vi "Breakfast Menu W3.vi"() -> ()   [LabVIEW 2019, in "Tree Map.lvlib"]
doc: "<b>Author:</b> Piotr Kruczkowski <PrimaryKey>\n<b>License:</b> NewBSD\n\nCopyright (c) 2019, National Instruments\nAll rights reserved.\n\nRedistribution and use in source and binary forms, with or without\nmodification, are permitted provided that the following conditions are met:\n1. Redistributions of source code must retain the above copyright\n notice, this list of conditions and the following disclaimer.\n2. Redistributions in binary form must reproduce the above copyright\n notice, this list of conditions and the following disclaimer in the\n documentation and/or other materials provided with the distribution.\n3. Neither the name of National Instruments nor the\n names of its contributors may be used to endorse or promote products\n derived from this software without specific prior written permission.\n\nTHIS SOFTWARE IS PROVIDED BY National Instruments ''AS IS'' AND ANY\nEXPRESS OR IMPLIED WARRANTIES, INCLUDING, BUT NOT LIMITED TO, THE IMPLIED\nWARRANTIES OF MERCHANTABILITY AND FITNESS FOR A PARTICULAR PURPOSE ARE\nDISCLAIMED. IN NO EVENT SHALL National Instruments BE LIABLE FOR ANY\nDIRECT, INDIRECT, INCIDENTAL, SPECIAL, EXEMPLARY, OR CONSEQUENTIAL DAMAGES\n(INCLUDING, BUT NOT LIMITED TO, PROCUREMENT OF SUBSTITUTE GOODS OR SERVICES;\nLOSS OF USE, DATA, OR PROFITS; OR BUSINESS INTERRUPTION) HOWEVER CAUSED AND\nON ANY THEORY OF LIABILITY, WHETHER IN CONTRACT, STRICT LIABILITY, OR TORT\n(INCLUDING NEGLIGENCE OR OTHERWISE) ARISING IN ANY WAY OUT OF THE USE OF THIS\nSOFTWARE, EVEN IF ADVISED OF THE POSSIBILITY OF SUCH DAMAGE."
uses:
  Tree Map.lvlib
  Tree Map Data.ctl
  API/List Roots.vi
  Utility/Into Tree Control Items.vi
panel:
  out "Tree Map":T1={"\\breakfast_menu"={"Child Paths Set"={"\\breakfast_menu\\food", "\\breakfast_menu\\food_000000", "\\breakfast_menu\\food_000001", "\\breakfast_menu\\food_000002", "\\breakfast_menu\\food_000003"}, "Name"="breakfast_menu", "Data"="", "Attributes"={}}, "\\breakfast_menu\\food"={"Child Paths Set"={"\\breakfast_menu\\food\\calories", "\\breakfast_menu\\food\\description", "\\breakfast_menu\\food\\name", "\\breakfast_menu\\food\\price"}, "Name"="food", "Data"="", "Attributes"={}}, "\\breakfast_menu\\food\\calories"={"Child Paths Set"={}, "Name"="calories", "Data"="650", "Attributes"={}}, "\\breakfast_menu\\food\\description"={"Child Paths Set"={}, "Name"="description", "Data"="Two of our famous Belgian Waffles with plenty of real maple syrup", "Attributes"={}}, "\\breakfast_menu\\food\\name"={"Child Paths Set"={}, "Name"="name", "Data"="Belgian Waffles", "Attributes"={}}, "\\breakfast_menu\\food\\price"={"Child Paths Set"={}, "Name"="price", "Data"="$5.95", "Attributes"={}}, "\\breakfast_menu\\food_000000"={"Child Paths Set"={"\\breakfast_menu\\food_000000\\calories", "\\breakfast_menu\\food_000000\\description", "\\breakfast_menu\\food_000000\\name", "\\breakfast_menu\\food_000000\\price"}, "Name"="food", "Data"="", "Attributes"={}}, "\\breakfast_menu\\food_000000\\calories"={"Child Paths Set"={}, "Name"="calories", "Data"="900", "Attributes"={}}, "\\breakfast_menu\\food_000000\\description"={"Child Paths Set"={}, "Name"="description", "Data"="Light Belgian waffles covered with strawberries and whipped cream", "Attributes"={}}, "\\breakfast_menu\\food_000000\\name"={"Child Paths Set"={}, "Name"="name", "Data"="Strawberry Belgian Waffles", "Attributes"={}}, "\\breakfast_menu\\food_000000\\price"={"Child Paths Set"={}, "Name"="price", "Data"="$7.95", "Attributes"={}}, "\\breakfast_menu\\food_000001"={"Child Paths Set"={"\\breakfast_menu\\food_000001\\calories", "\\breakfast_menu\\food_000001\\description", "\\breakfast_menu\\food_000001\\name", "\\breakfast_menu\\food_000001\\price"}, "Name"="food", "Data"="", "Attributes"={}}, "\\breakfast_menu\\food_000001\\calories"={"Child Paths Set"={}, "Name"="calories", "Data"="900", "Attributes"={}}, "\\breakfast_menu\\food_000001\\description"={"Child Paths Set"={}, "Name"="description", "Data"="Light Belgian waffles covered with an assortment of fresh berries and whipped cream", "Attributes"={}}, "\\breakfast_menu\\food_000001\\name"={"Child Paths Set"={}, "Name"="name", "Data"="Berry-Berry Belgian Waffles", "Attributes"={}}, "\\breakfast_menu\\food_000001\\price"={"Child Paths Set"={}, "Name"="price", "Data"="$8.95", "Attributes"={}}, "\\breakfast_menu\\food_000002"={"Child Paths Set"={"\\breakfast_menu\\food_000002\\calories", "\\breakfast_menu\\food_000002\\description", "\\breakfast_menu\\food_000002\\name", "\\breakfast_menu\\food_000002\\price"}, "Name"="food", "Data"="", "Attributes"={}}, "\\breakfast_menu\\food_000002\\calories"={"Child Paths Set"={}, "Name"="calories", "Data"="600", "Attributes"={}}, "\\breakfast_menu\\food_000002\\description"={"Child Paths Set"={}, "Name"="description", "Data"="Thick slices made from our homemade sourdough bread", "Attributes"={}}, "\\breakfast_menu\\food_000002\\name"={"Child Paths Set"={}, "Name"="name", "Data"="French Toast", "Attributes"={}}, "\\breakfast_menu\\food_000002\\price"={"Child Paths Set"={}, "Name"="price", "Data"="$4.50", "Attributes"={}}, "\\breakfast_menu\\food_000003"={"Child Paths Set"={"\\breakfast_menu\\food_000003\\calories", "\\breakfast_menu\\food_000003\\description", "\\breakfast_menu\\food_000003\\name", "\\breakfast_menu\\food_000003\\price"}, "Name"="food", "Data"="", "Attributes"={}}, "\\breakfast_menu\\food_000003\\calories"={"Child Paths Set"={}, "Name"="calories", "Data"="950", "Attributes"={}}, "\\breakfast_menu\\food_000003\\description"={"Child Paths Set"={}, "Name"="description", "Data"="Two eggs, bacon or sausage, toast, and our ever-popular hash browns", "Attributes"={}}, "\\breakfast_menu\\food_000003\\name"={"Child Paths Set"={}, "Name"="name", "Data"="Homestyle Breakfast", "Attributes"={}}, "\\breakfast_menu\\food_000003\\price"={"Child Paths Set"={}, "Name"="price", "Data"="$6.95", "Attributes"={}}}
  in  "Tree Control":string(tree)
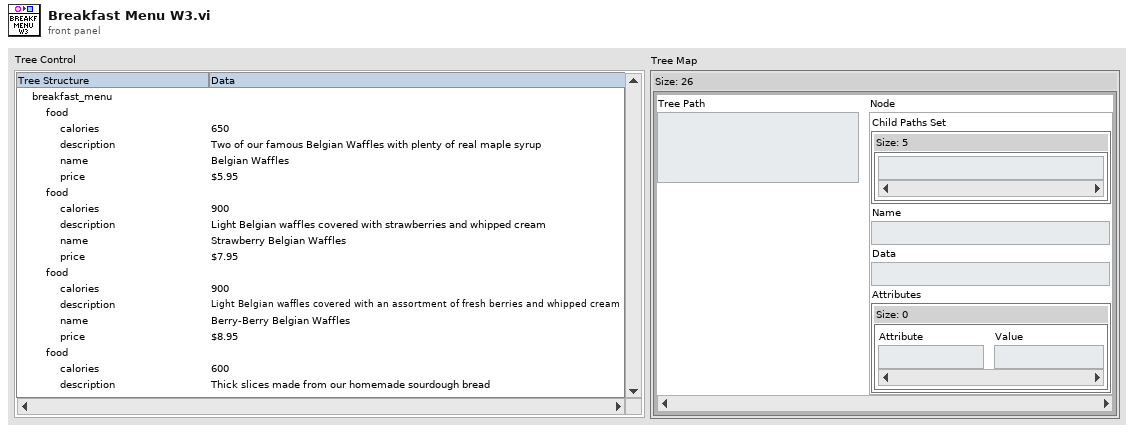
[diagram p1: front panel]
types:
  T1 = typedef "Tree Map.lvlib/Tree Map Data.ctl" = map{string, cluster{"Child Paths Set":set{string}, "Name":string, "Data":string, "Attributes":map{string, string}}}
  T2 = cluster{"Left Cell String":string, "Child Text":string[], "Child Tag":string, "Item Indent":i32, "Child Only?":bool, "Glyph Index":i32}[]
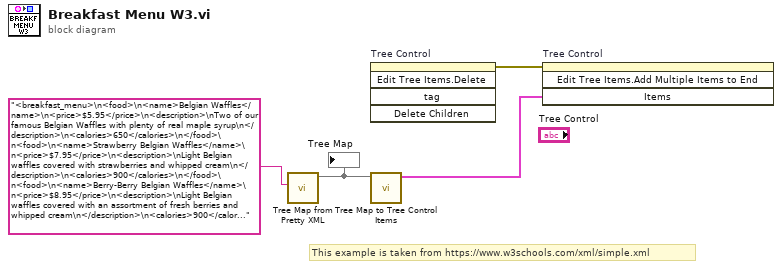
[diagram p0: block diagram]
diagram:
  # "This example is taken from https://www.w3schools.com/xml/simple.xml"
  n1 = call "Tree Map from Pretty XML.vi"("Pretty XML"="<breakfast_menu>\n<food>\n<name>Belgian Waffles</name>\n<price>$5.95</price>\n<description>\nTwo of our famous Belgian Waffles with plenty of real maple syrup\n</description>\n<calories>650</calories>\n</food>\n<food>\n<name>Strawberry Belgian Waffles</name>\n<price>$7.95</price>\n<description>\nLight Belgian waffles covered with strawberries and whipped cream\n</description>\n<calories>900</calories>\n</food>\n<food>\n<name>Berry-Berry Belgian Waffles</name>\n<price>$8.95</price>\n<description>\nLight Belgian waffles covered with an assortment of fresh berries and whipped cream\n</description>\n<calories>900</calories>\n</food>\n<food>\n<name>French Toast</name>\n<price>$4.50</price>\n<description>\nThick slices made from our homemade sourdough bread\n</description>\n<calories>600</calories>\n</food>\n<food>\n<name>Homestyle Breakfast</name>\n<price>$6.95</price>\n<description>\nTwo eggs, bacon or sausage, toast, and our ever-popular hash browns\n</description>\n<calories>950</calories>\n</food>\n</breakfast_menu>") -> ("Tree Map Out"=w3:T1)  [unwired: 9 in, 1 out]
  "Tree Map" <- w3
  n2 = invoke on="Tree Control" class="Tree (strict)" method="Edit Tree Items.Delete"() -> (error out=w4:errorcluster)  [unwired: 5 in, 4 out]
  n3 = call "Tree Map to Tree Control Items.vi"("Tree Map In"=w3) -> ("Tree Control Items"=w2:T2)  [unwired: 10 in]
  n4 = invoke on="Tree Control" class="Tree (strict)" method="Edit Tree Items.Add Multiple Items to End"(error in=w4, "Items"=w2) -> ()  [unwired: 2 in, 4 out]
